vi "Add Analog Replay.vi"(8 "error in (no error)":errorcluster, 9 "Analog Replay Data Options":T1={"Input file"=path "", "Group"="", "Channel"="", "Reverse"=FALSE, "FPGA Memory Size"=enum."16,384", "Position reference"=enum."Crank angle", "Data selection method"=enum."Manual", "Offset"=0, "Samples"=0, "Missing teeth location"=0.0, "DataPlugin"=""}, 10 "Analog Replay Settings":T5={"Name"="", "DAC bipolar range (V)"=10.0, "Voltage below min speed"=0.0, "Min speed (RPM)"=0.0, "Voltage at min speed"=0.0, "Max speed (RPM)"=10000.0, "Voltage at max speed"=10.0, "Negate playback voltage values at negative engine speed"=TRUE, "Allow run-time override of voltage scaling"=FALSE}, 11 "APU Node in":refnum<k24>) -> (0 "error out":errorcluster, 2 "Analog Replay out":refnum<k24>, 3 "APU Node out":refnum<k24>)   [LabVIEW 2015, in "Engine Simulation Toolkit SysDef API.lvlib"]
uses:
  Engine Simulation Toolkit SysDef API.lvlib
  Analog Replay Settings.ctl
  NationalInstruments.VeriStand.SystemDefinitionAPI
  Analog Replay Data Options.ctl
  System Explorer/FPGA Mem Size.ctl
  System Explorer/Position Reference.ctl
  System Explorer/Data Replay Data Selection Method.ctl
  System Explorer/Engine Simulation Toolkit System Explorer.lvlib
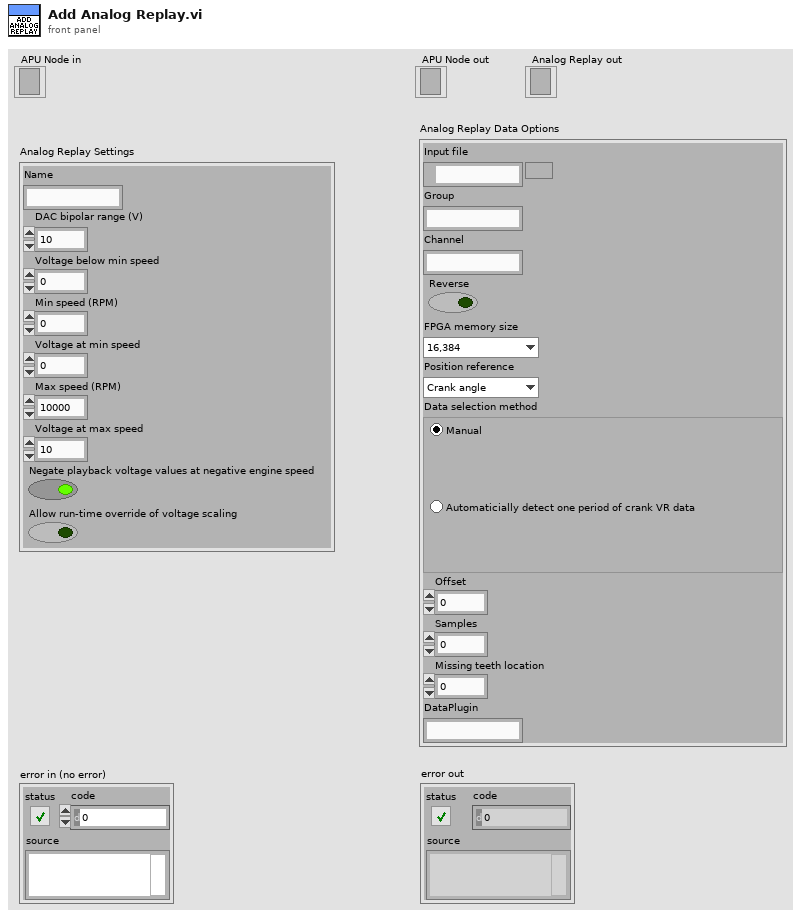
[diagram p1: front panel]
types:
  T1 = typedef "Engine Simulation Toolkit SysDef API.lvlib/Analog Replay Data Options.ctl" = cluster{"Input file":path, "Group":string, "Channel":string, "Reverse":bool, "FPGA Memory Size":T2, "Position reference":T3, "Data selection method":T4, "Offset":i32, "Samples":i32, "Missing teeth location":dbl, "DataPlugin":string}
  T2 = typedef "Engine Simulation Toolkit System Explorer.lvlib/FPGA Mem Size.ctl" = enum16{"65,536", "32,768", "16,384", "8,192", "4,096", "2,048", "1,024"}
  T3 = typedef "Engine Simulation Toolkit System Explorer.lvlib/Position Reference.ctl" = enum16{"Crank angle", "Cycle angle"}
  T4 = typedef "Engine Simulation Toolkit System Explorer.lvlib/Data Replay Data Selection Method.ctl" = enum32{"Manual", "AutoVRCrank"}
  T5 = typedef "Engine Simulation Toolkit SysDef API.lvlib/Analog Replay Settings.ctl" = cluster{"Name":string, "DAC bipolar range (V)":dbl, "Voltage below min speed":dbl, "Min speed (RPM)":dbl, "Voltage at min speed":dbl, "Max speed (RPM)":dbl, "Voltage at max speed":dbl, "Negate playback voltage values at negative engine speed":bool, "Allow run-time override of voltage scaling":bool}
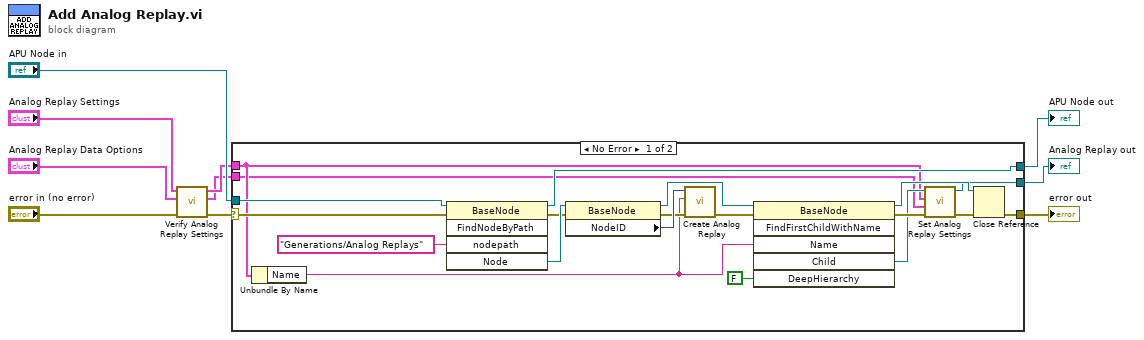
[diagram p0: block diagram]
diagram:
  n1 = call "Verify Analog Replay Settings.vi"("error in (no error)"="error in (no error)", "Analog Replay Data Options in"="Analog Replay Data Options", "Analog Replay Settings in"="Analog Replay Settings") -> ("error out"=w6:errorcluster, "Analog Replay Data Options out"=w2:T1, "Analog Replay Settings out"=w4:T5)  [unwired: 6 in]
  n2 = case shown="No Error" w6 {
    selector: w6 -> [w25 w32]
    tunnel: "APU Node in" -> [w27 w31]
    tunnel: [w23 w31] -> w9
    tunnel: [w22 w32] -> w8
    tunnel: w4 -> [w12 _]
    tunnel: w2 -> [w11 _]
    tunnel: [w13 _] -> w1
    frame No Error {
      n3 = Unbundle By Name(w12) -> ("Name"=w18:string)
      n4 = invoke class="BaseNode" method="FindNodeByPath"(reference=w27, error in=w25, "nodepath"="Generations/Analog Replays") -> (reference out=w23:refnum<k24>, error out=w24:errorcluster, "Node"=w26:refnum<k24>)  [unwired: 2 in, 2 out]
      n5 = property class="BaseNode"(reference=w26, error in=w24) -> (reference out=w20:refnum<k24>, error out=w29:errorcluster, "NodeID"=w30:u64)
      n6 = call "Create Analog Replay.vi"("error in (no error)"=w29, "analog replay name"=w18, "Section Ptr"=w30) -> ("error out"=w28:errorcluster)  [unwired: 6 in, 2 out]
      n7 = invoke class="BaseNode" method="FindFirstChildWithName"(reference=w20, error in=w28, "Name"=w18, "DeepHierarchy"=FALSE) -> (reference out=w19:refnum<k24>, error out=w16:errorcluster, "Child"=w14:refnum<k24>)  [unwired: 2 in, 3 out]
      n8 = call "Set Analog Replay Settings.vi"("error in (no error)"=w16, "Analog Replay Data Options"=w11, "Analog Replay Settings"=w12, "Analog Replay in"=w14) -> ("error out"=w15:errorcluster, "Analog Replay out"=w13:refnum<k24>)  [unwired: 6 in]
      n9 = Close Reference(reference=w19, error in (no error)=w15) -> (error out=w22:errorcluster)
    }
    frame Error {
    }
  }
  "APU Node out" <- w9
  "error out" <- w8
  "Analog Replay out" <- w1
